vi "GPIB Numbers.vi"() -> ()   [LabVIEW 2009]
uses:
  GPIB Type Def.ctl
  Instruments/Magnet/Oxford/PSSUBS.LLB/PSIO.ctl
  Instruments/Magnet/Oxford/BUSGEN.LLB/OxfordAddress.ctl
  Instruments/Magnet/Oxford/ITCSUBS.LLB/ITCIO.ctl
  Instruments/Magnet/Oxford/ITCSUBS.LLB/ITCVersion.ctl
  USBMono Type Def.ctl
  USBCCD Type Def.ctl
panel:
  in  "Microwave Amplifier":T1={"Name"="Microwave Gen.", "bus"=0.0, "GPIB"=19.0, "GPIB as string"="19", "byte"=1024, "VISA Resource Name"="GPIB0::19::INSTR"}
  in  "Synapse CCD":T2={"Name"="Synapse CCD", "Unique ID"="CCD1", "Mono Unique ID"="Mono1"}
  in  "iHR 320 Spectrometer":T3={"Name"="iHR 320 Spectr.", "Unique ID"="Mono2", "FW Unique ID"="FW1"}
  in  "Laser Power Controller":T1={"Name"="LPC", "bus"=0.0, "GPIB"=3.0, "GPIB as string"="3", "byte"=1024, "VISA Resource Name"="GPIB0::3::INSTR"}
  in  "Power Meter":T1={"Name"="Power Meter", "bus"=0.0, "GPIB"=4.0, "GPIB as string"="4", "byte"=1024, "VISA Resource Name"="GPIB0::4::INSTR"}
  in  "Oxford Temperature Controller":T4={"Address"={"Com Port"=1, "ISOBUS Address"=1, "GPIB Address"=24, "Communication"=enum."ISOBUS"}, "Version"=enum."ITC503", "Ch 1 dec places"=1, "Ch 2 dec places"=1, "Ch 3 dec places"=1, "Ch1 Name"="Temperature", "Ch2 Name"="", "Ch3 Name"=""}
  in  "Oxford Level Meter":T7={"Address"={"Com Port"=1, "ISOBUS Address"=5, "GPIB Address"=24, "Communication"=enum."ISOBUS"}, "ILM Name"="", "Display Channel"=[]}
  in  "Oxford Power Supply":T8={"Address"={"Com Port"=1, "ISOBUS Address"=2, "GPIB Address"=25, "Communication"=enum."ISOBUS"}, "Version"=enum."IPS"}
  in  "Borrowed Lockin SR830":T1={"Name"="Borrowed Lockin SR830", "bus"=0.0, "GPIB"=7.0, "GPIB as string"="7", "byte"=1024, "VISA Resource Name"="GPIB0::7::INSTR"}
  in  "Lockin SR810":T1={"Name"="Lockin SR810", "bus"=0.0, "GPIB"=8.0, "GPIB as string"="8", "byte"=1024, "VISA Resource Name"="GPIB0::8::INSTR"}
  in  "Fluke Multimeter":T1={"Name"="Fluke Multimeter", "bus"=0.0, "GPIB"=2.0, "GPIB as string"="2", "byte"=0, "VISA Resource Name"="GPIB0::2::INSTR"}
  in  "Digikrom Spectrometer":T1={"Name"="Digikrom Spectr.", "bus"=0.0, "GPIB"=0.0, "GPIB as string"="0", "byte"=0, "VISA Resource Name"="COM1"}
  in  "Oxford Magnet":T1={"Name"="Oxford Magnet", "bus"=0.0, "GPIB"=0.0, "GPIB as string"="0", "byte"=0, "VISA Resource Name"="COM1"}
  in  "Translation Stage":T1={"Name"="Translation Stage", "bus"=0.0, "GPIB"=6.0, "GPIB as string"="6", "byte"=1024, "VISA Resource Name"="GPIB0::6::INSTR"}
  in  "DAQ / Analog":cluster{"DAQmx Task Name":refnum<k21>}={"DAQmx Task Name"="Analog Channels 0-1"}
  in  "FG":T1={"Name"="Function Gen.", "bus"=0.0, "GPIB"=11.0, "GPIB as string"="11", "byte"=1024, "VISA Resource Name"="AFG3252"}
  in  "Microwave":T1={"Name"="Microwave Gen.", "bus"=0.0, "GPIB"=19.0, "GPIB as string"="19", "byte"=1024, "VISA Resource Name"="GPIB0::19::INSTR"}
  in  "JY Spectrometer":T1={"Name"="JY Spectrometer", "bus"=0.0, "GPIB"=1.0, "GPIB as string"="1", "byte"=1024, "VISA Resource Name"="GPIB0::1::INSTR"}
  in  "Lockin SR830":T1={"Name"="Lockin SR830", "bus"=0.0, "GPIB"=9.0, "GPIB as string"="9", "byte"=1024, "VISA Resource Name"="GPIB0::9::INSTR"}
  in  "PG":T1={"Name"="Pulse Generator", "bus"=0.0, "GPIB"=10.0, "GPIB as string"="10", "byte"=1024, "VISA Resource Name"="GPIB0::10::INSTR"}
  in  "PC":T1={"Name"="Photon Counter", "bus"=0.0, "GPIB"=23.0, "GPIB as string"="23", "byte"=1024, "VISA Resource Name"="GPIB0::23::INSTR"}
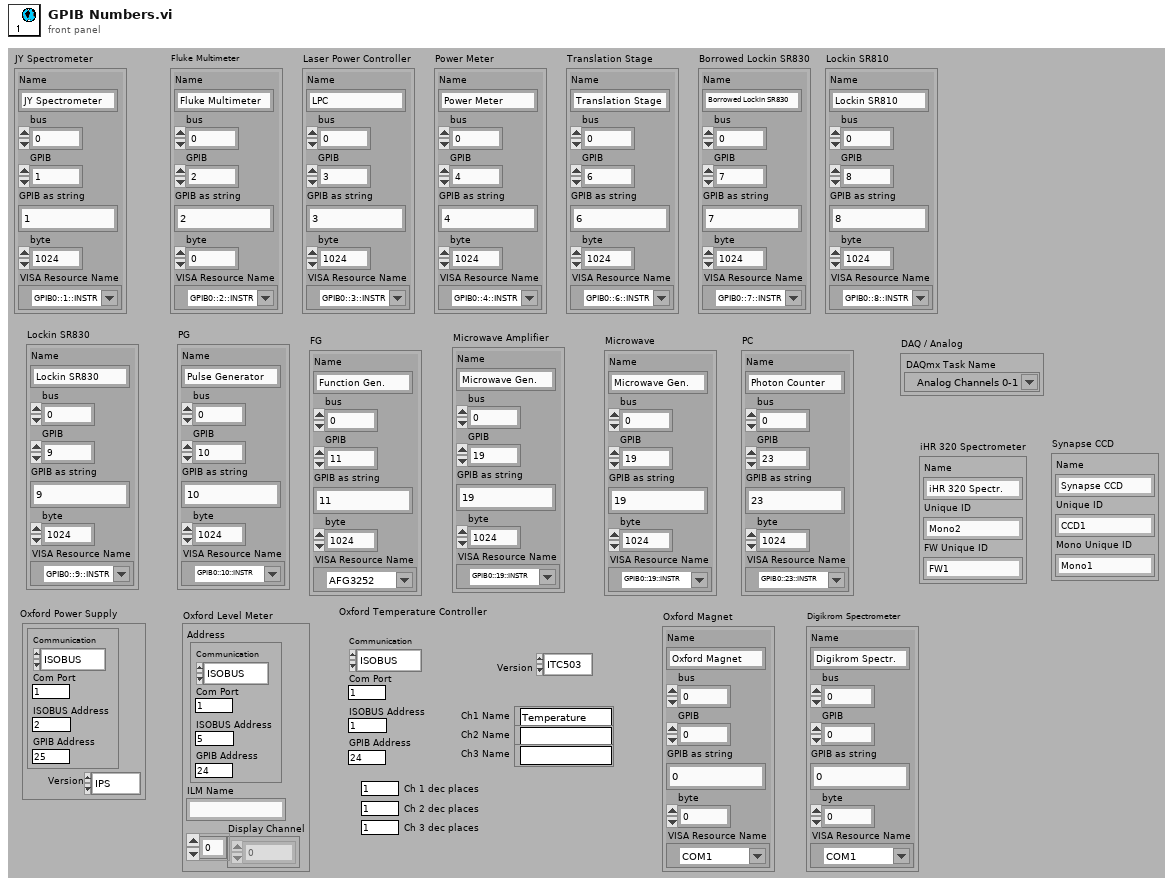
[diagram p1: front panel]
types:
  T1 = typedef "GPIB Type Def.ctl" = cluster{"Name":string, "bus":dbl, "GPIB":dbl, "GPIB as string":string, "byte":i32, "VISA Resource Name":refnum<visa-resource-name>}
  T2 = typedef "USBCCD Type Def.ctl" = cluster{"Name":string, "Unique ID":string, "Mono Unique ID":string}
  T3 = typedef "USBMono Type Def.ctl" = cluster{"Name":string, "Unique ID":string, "FW Unique ID":string}
  T4 = typedef "ITCIO.ctl" = cluster{"Address":T5, "Version":T6, "Ch 1 dec places":i16, "Ch 2 dec places":i16, "Ch 3 dec places":i16, "Ch1 Name":string, "Ch2 Name":string, "Ch3 Name":string}
  T5 = typedef "OxfordAddress.ctl" = cluster{"Com Port":i32, "ISOBUS Address":i32, "GPIB Address":i16, "Communication":enum16{"RS232", "ISOBUS", "GPIB", "Gateway"}}
  T6 = typedef "ITCVersion.ctl" = enum16{"ITC502", "ITC503", "ITC601"}
  T7 = cluster{"Address":T5, "ILM Name":string, "Display Channel":i32[]}
  T8 = typedef "PSIO.ctl" = cluster{"Address":T5, "Version":enum16{"PS", "IPS"}}
diagram:
